vi "SeqMgr.Test Reset.vi"(8 "error in (no error)":errorcluster, 11 "SeqMgr in":refnum<class "SeqMgr.lvclass">) -> (0 "error out":errorcluster, 3 "SeqMgr out":refnum<class "SeqMgr.lvclass">)   [LabVIEW 2024, in "EQMF.lvlib" / "SeqMgr.lvlib" / "SeqMgr.lvclass"]
uses:
  SeqMgr.lvclass
  SeqMgr.Result Info.ctl
  SeqMgr.Result State Enum.ctl
  SeqMgr.Progress Info.ctl
  SeqMgr.Progress Type.ctl
  Queues/Q.Msg Return Info.ctl
  Queues/Q.Element.ctl
  SeqMgr.lvclass/SeqMgr.ctl
  SeqMgr.lvlib
  Queues/Queue Utils.lvlib
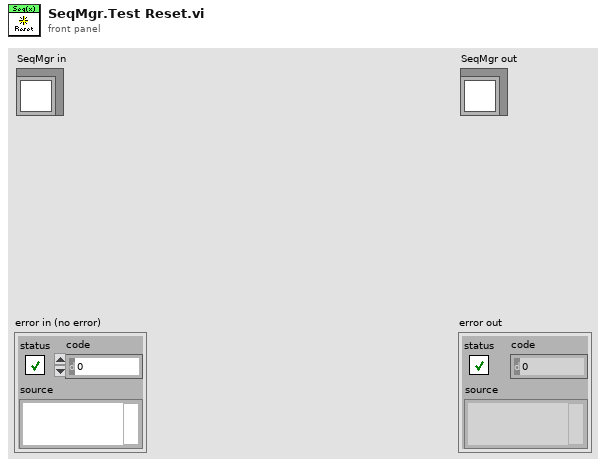
[diagram p1: front panel]
types:
  T1 = typedef "EQMF.lvlib/Queue Utils.lvlib/Q.Msg Return Info.ctl" = cluster{"Ret Q":refnum<queue>, "Ret Msg":T2, "SeqNum":i32}
  T2 = typedef "EQMF.lvlib/Queue Utils.lvlib/Q.Element.ctl" = cluster{"Cmd":string, "Sub":string, "Data1":variant, "Data2":variant}
  T3 = typedef "EQMF.lvlib/SeqMgr.lvlib/SeqMgr.Progress Info.ctl" = cluster{"Running":bool, "StartTime":timestamp, "EndTime":timestamp, "Progress":dbl, "Duration(s)":dbl, "ProgType":T4, "StepCnt":i32, "StepTotal":i32, "RemainingTime(s)":dbl, "Test State":enum32{"Idle", "Running", "Completed"}}
  T4 = typedef "EQMF.lvlib/SeqMgr.lvlib/SeqMgr.Progress Type.ctl" = enum16{"Steps", "Time"}
  T5 = typedef "EQMF.lvlib/SeqMgr.lvlib/SeqMgr.Result Info.ctl" = cluster{"State":T6, "Code":i32, "Description":string}
  T6 = typedef "EQMF.lvlib/SeqMgr.lvlib/SeqMgr.Result State Enum.ctl" = enum16{"None", "Passing", "Failing", "PASS", "FAIL", "ABORT", "ERROR"}
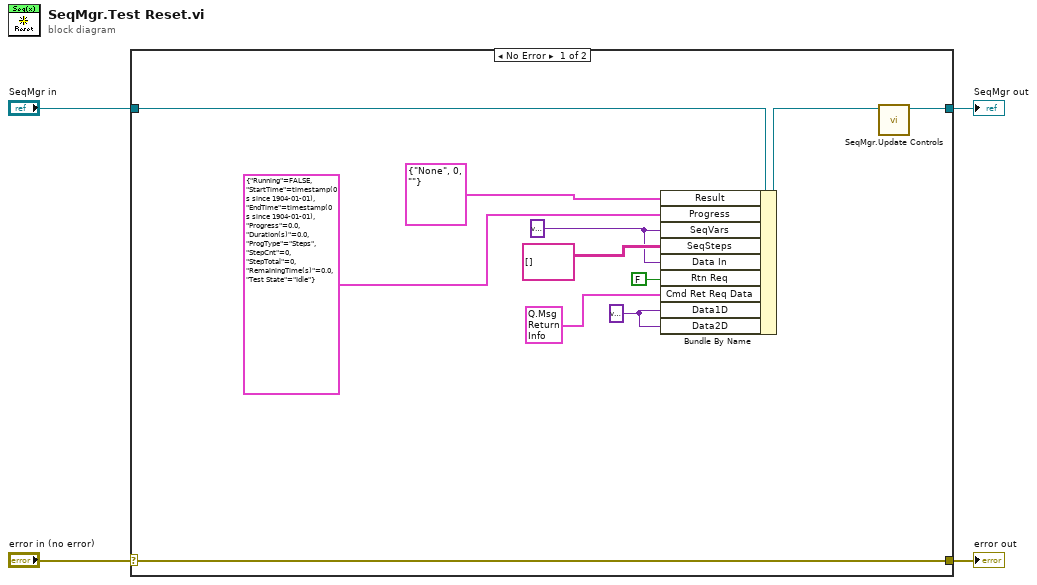
[diagram p0: block diagram]
diagram:
  n1 = case shown="No Error" "error in (no error)" {
    selector: "error in (no error)" -> [w15 w17]
    tunnel: [w15 w17] -> w3
    tunnel: [w12 w16] -> w1
    tunnel: "SeqMgr in" -> [w14 w16]
    frame No Error {
      w5 = variant ("Data1D")
      w8 = variant ("SeqVars")
      n2 = Bundle By Name(cluster=w14, "Result"=T5 {"State"=enum."None", "Code"=0, "Description"=""}, "Progress"=T3 {"Running"=FALSE, "StartTime"=timestamp(0 s since 1904-01-01), "EndTime"=timestamp(0 s since 1904-01-01), "Progress"=0.0, "Duration(s)"=0.0, "ProgType"=enum."Steps", "StepCnt"=0, "StepTotal"=0, "RemainingTime(s)"=0.0, "Test State"=enum."Idle"}, "SeqVars"=w8, "SeqSteps"=string[][] [], "Data In"=w8, "Rtn Req"=FALSE, "Cmd Ret Req Data"=T1 {"Ret Q"=refnum, "Ret Msg"={"Cmd"="", "Sub"="", "Data1"=variant, "Data2"=variant}, "SeqNum"=0}, "Data1D"=w5, "Data2D"=w5) -> (w13:refnum<class "SeqMgr.lvclass">)
      n3 = call "SeqMgr.Update Controls.vi"("SeqMgr in"=w13) -> ("SeqMgr out"=w12:refnum<class "SeqMgr.lvclass">)  [unwired: 9 in, 1 out]
    }
    frame Error {
    }
  }
  "error out" <- w3
  "SeqMgr out" <- w1
